vi "Covariance Matrix.vi"(11 "X":dbl[][](array[numeric])) -> (2 "mean vector":dbl[](array[numeric]), 3 "covariance matrix V":T1)   [LabVIEW 2020, in "NI_Gmath.lvlib"]
doc: "Computes the covariance matrix of the input sequence <B>X</B>."
uses:
  NI_Gmath.lvlib
  RealMatrix.ctl
  NI_AALBase.lvlib
  NI_Matrix.lvlib
panel:
  # "Covariance Matrix"
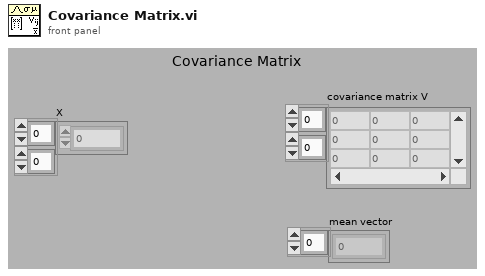
[diagram p1: front panel]
types:
  T1 = typedef "NI_Matrix.lvlib/RealMatrix.ctl" = dbl[][]
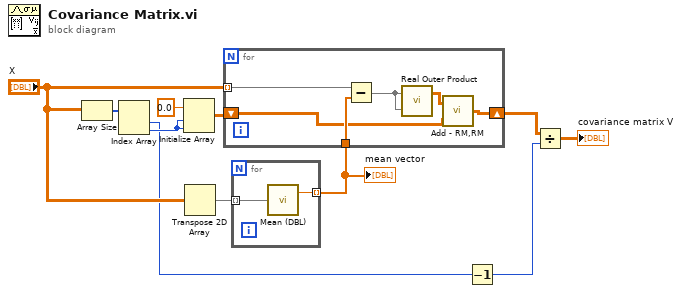
[diagram p0: block diagram]
diagram:
  n1 = Array Size(array="X") -> (size(s)=w7:i32[])
  n2 = Index Array(array=w7) -> (element #1=w4:i32, element #2=w5:i32)  [unwired: 2 in]
  n3 = Initialize Array(0.0 ("element"), w5, w5) -> (w9:dbl[][])
  n4 = Transpose 2D Array(2D array="X") -> (transposed array=w11:dbl[][])
  n5 = for {
    tunnel: w11 -> [w13] mode=indexing
    tunnel: [w12] -> w10 mode=indexing
    n6 = call "Mean (DBL).vi"("X"=w13) -> ("mean"=w12:dbl)  [unwired: 1 out]
  }
  "mean vector" <- w10
  n7 = for {
    tunnel: "X" -> [w18] mode=indexing
    tunnel: w10 -> [w19]
    shift-right: [w14] -> w3
    shift-left: w9 -> [w15]
    n8 = Subtract(x=w18, y=w19) -> (x-y=w17:dbl[])
    n9 = call "Real Outer Product.vi"("Y Vector"=w17, "X Vector"=w17) -> ("Outer Product"=w16:T1)  [unwired: 1 out]
    n10 = call "Add - RM,RM.vi"("Real Matrix B"=w15, "Real Matrix A"=w16) -> ("A + B"=w14:T1)
  }
  n11 = Decrement(x=w4) -> (x-1=w1:i32)
  n12 = Divide(x=w3, y=w1) -> (x/y=→"covariance matrix V":T1)
